vi "Knock Cylinder 1.0 Write Inputs.vi"(4 "Angle multiplier":dbl, 5 "Device inputs":dbl[](array[numeric]), 6 "DAC multiplier":dbl, 7 "Last Device inputs":dbl[](array[numeric]), 8 "error in (no error)":errorcluster, 9 "input reference in":T1, 10 "input in":T2, 11 "FIFO indexes.inputs":T3) -> (0 "error out":errorcluster, 1 "input reference out":T1, 2 "input out":T2)   [LabVIEW 2019, in "Engine Simulation Toolkit Engine.lvlib"]
uses:
  Engine Simulation Toolkit Engine.lvlib
  Shared/1.0 Knock Cylinder FIFO Idxs.ctl
  Knock Cylinder 1.0 Input Ref.ctl
  Shared/Engine Simulation Toolkit Shared.lvlib
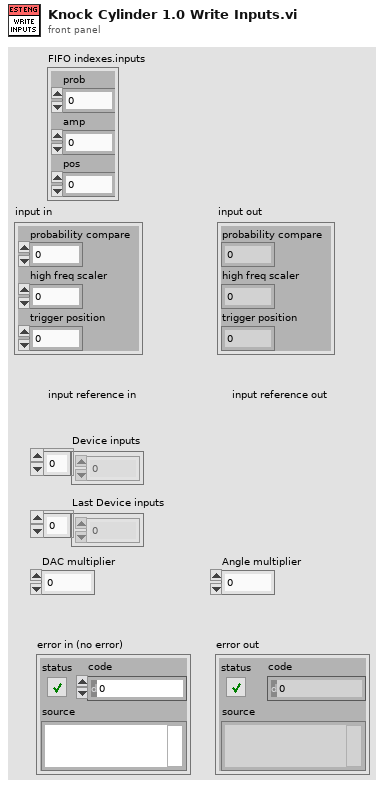
[diagram p1: front panel]
types:
  T1 = typedef "Engine Simulation Toolkit Engine.lvlib/Knock Cylinder 1.0 Input Ref.ctl" = refnum<k20>
  T2 = cluster{"probability compare":u16, "high freq scaler":fxp<+,10,0>, "trigger position":u16}
  T3 = typedef "Engine Simulation Toolkit Shared.lvlib/1.0 Knock Cylinder FIFO Idxs.ctl" = cluster{"prob":i32, "amp":i32, "pos":i32}
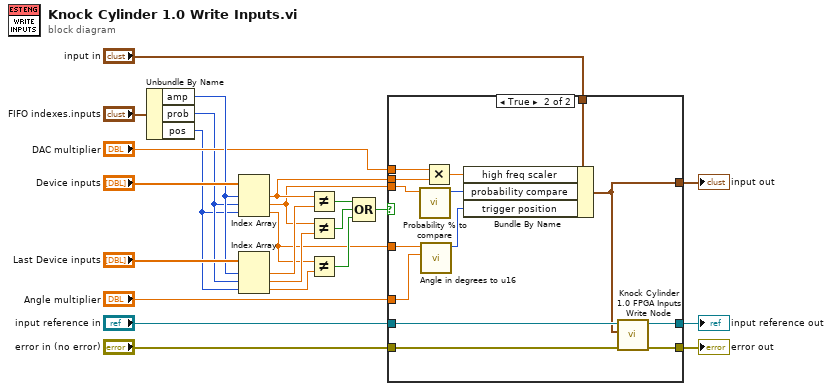
[diagram p0: block diagram]
diagram:
  n1 = Unbundle By Name("FIFO indexes.inputs") -> ("amp"=w16:i32, "prob"=w11:i32, "pos"=w6:i32)
  n2 = Index Array(array="Device inputs", index #1=w16, index #2=w11, index #3=w6) -> (element #1=w13:dbl, element #2=w8:dbl, element #3=w1:dbl)
  n3 = Index Array(array="Last Device inputs", index #1=w16, index #2=w11, index #3=w6) -> (element #1=w14:dbl, element #2=w9:dbl, element #3=w3:dbl)
  n4 = Not Equal?(x=w13, y=w14) -> (x != y?=w10:bool)
  n5 = Not Equal?(x=w8, y=w9) -> (x != y?=w5:bool)
  n6 = Not Equal?(x=w1, y=w3) -> (x != y?=w4:bool)
  n7 = Compound Arithmetic op=OR(w10, w5, w4) -> (w7:bool)
  n8 = case shown="True" w7 {
    tunnel: "error in (no error)" -> [w25 w41]
    tunnel: "input reference in" -> [w26 w40]
    tunnel: [w25 w39] -> w22
    tunnel: [w26 w38] -> w21
    tunnel: "input in" -> [w27 w37]
    tunnel: [w27 w36] -> w15
    tunnel: w13 -> [_ w35]
    tunnel: "DAC multiplier" -> [_ w34]
    tunnel: w8 -> [_ w32]
    tunnel: "Angle multiplier" -> [_ w30]
    tunnel: w1 -> [_ w28]
    frame False {
    }
    frame True {
      n9 = call "Probability % to compare.vi"("probability %"=w32) -> ("probability compare"=w31:u16)  [unwired: 10 in]
      n10 = call "Angle in degrees to u16.vi"("angle to u16 scale factor"=w30, "Angle (deg)"=w28) -> ("u16 angle"=w29:u16)  [unwired: 8 in, 1 out]
      n11 = Multiply(x=w34, y=w35) -> (x*y=w33:dbl)
      n12 = Bundle By Name(cluster=w37, "high freq scaler"=w33, "probability compare"=w31, "trigger position"=w29) -> (w36:T2)
      n13 = call "Knock Cylinder 1.0 FPGA Inputs Write Node.vi"("error in (no error)"=w41, "input"=w36, "Refnum in"=w40) -> ("error out"=w39:errorcluster, "Refnum out"=w38:T1)  [unwired: 7 in]
    }
  }
  "error out" <- w22
  "input out" <- w15
  "input reference out" <- w21
